vi "FPGA_R_ADC_W_DAC.vi"() -> ()   [LabVIEW 2019]
uses:
  <vilib>/rvi/Emulation/niFpgaGetClockAttributes.vi
  <vilib>/rvi/Emulation/niFpgaSctlEmulationGetInTimedLoop.vi
  <vilib>/rvi/Emulation/niFpgaEmulationReportErrorSimple.vi
  <vilib>/rvi/eio/common/nirviEmuTemplateMethod_errors.vi
  <vilib>/rvi/Emulation/niFpgaCriticalErrorInLSC.vi
  <vilib>/eio/EIONode/EIONode.xnode
panel:
  out "num refs":i16
  out "Tick Count(Ticks)":u32 caption="Encoder loop ticks"
  out "Encoder B Ref":bool
  out "Encoder A Ref":bool
  out "Encoder B":i32
  out "Encoder A":i32
  in  "stop 2":bool
  in  "Count(Ticks)":u32=800
  out "Data array":bool[](array[boolean])
  in  "stop":bool
  in  "DAC 3 write":bool[](array[boolean])=[FALSE, FALSE, FALSE, FALSE, FALSE, FALSE, FALSE, FALSE, FALSE, FALSE, FALSE, FALSE, FALSE, FALSE, FALSE, FALSE]
  in  "DAC 2 write":bool[](array[boolean])=[FALSE, FALSE, FALSE, FALSE, FALSE, FALSE, FALSE, FALSE, FALSE, FALSE, FALSE, FALSE, FALSE, FALSE, FALSE, FALSE]
  in  "DAC 1 write":bool[](array[boolean])=[FALSE, FALSE, FALSE, FALSE, FALSE, FALSE, FALSE, FALSE, FALSE, FALSE, FALSE, FALSE, FALSE, FALSE, FALSE, FALSE]
  out "ADC read":bool[](array[boolean])
  in  "ADC write":bool[](array[boolean])=[FALSE, FALSE, FALSE, FALSE, FALSE, TRUE, FALSE, FALSE, FALSE, FALSE, FALSE, FALSE, FALSE, FALSE, FALSE, FALSE]
  in  "Stop":bool
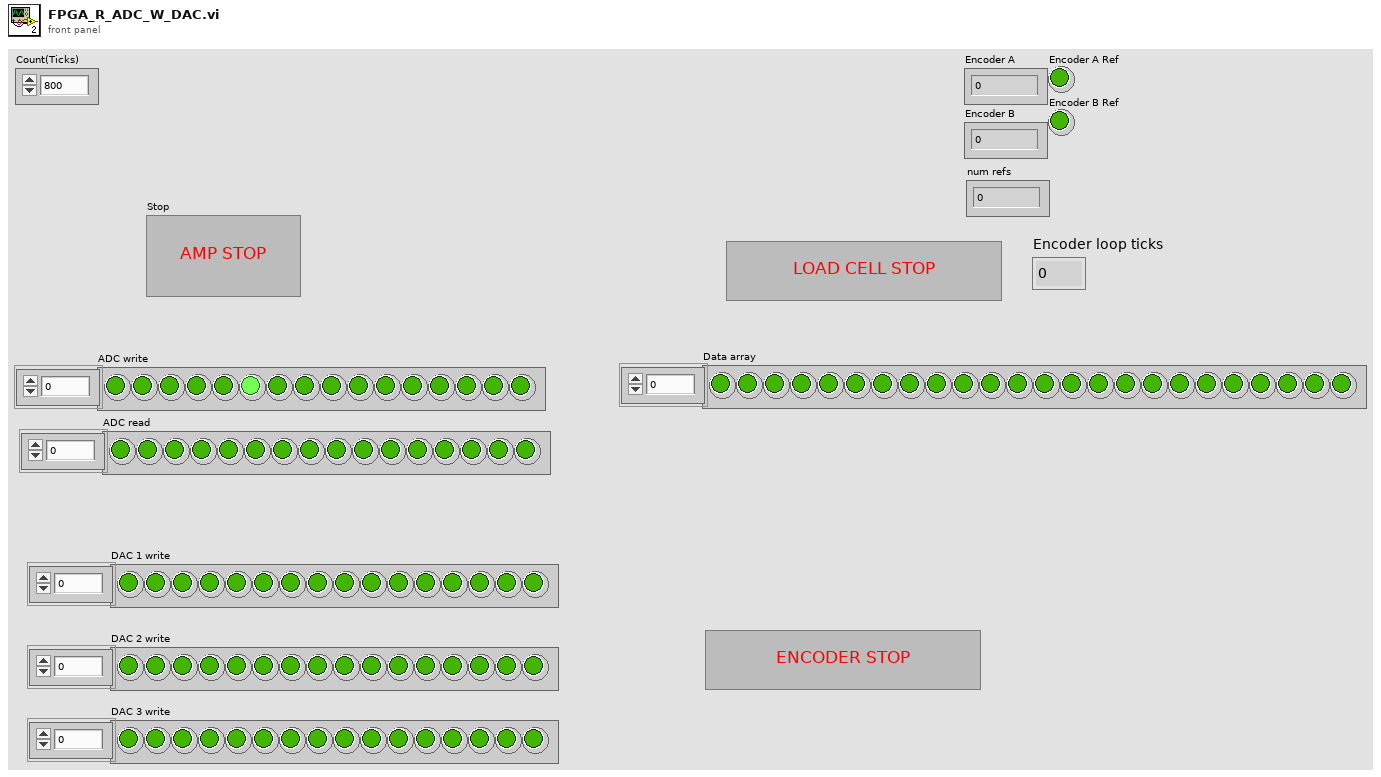
[diagram p1: front panel]
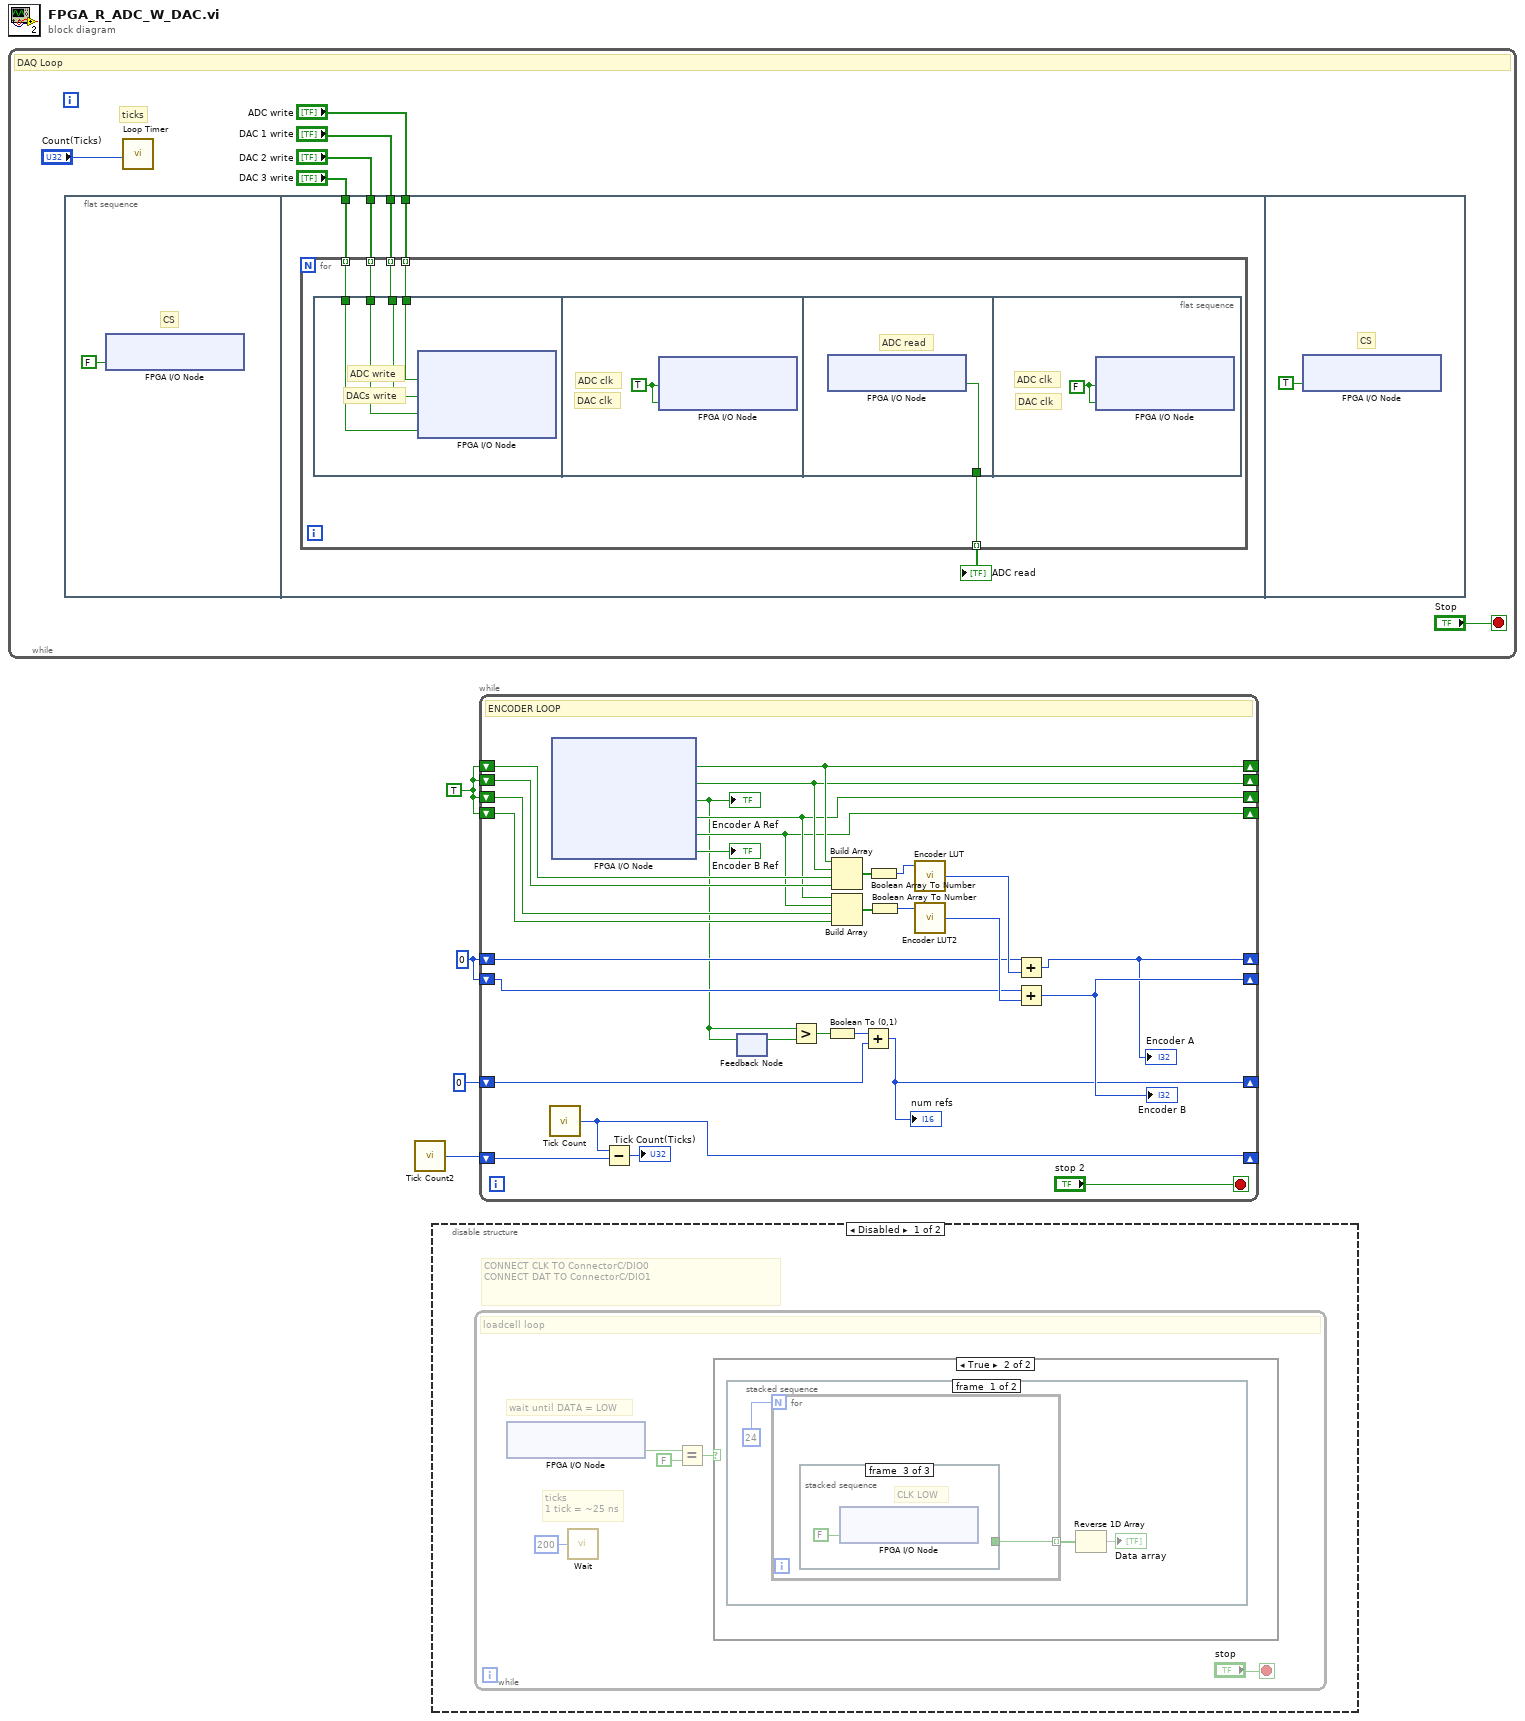
[diagram p0: block diagram]
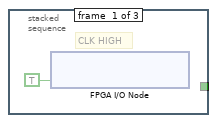
[diagram p3: hidden frame]
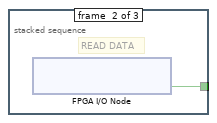
[diagram p4: hidden frame]
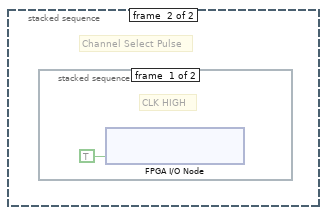
[diagram p5: hidden frame]
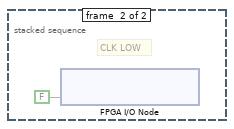
[diagram p6: hidden frame]
diagram:
  w3 = TRUE
  w4 = 0
  n1 = while {
    stop <- "Stop" stop-if-true
    # "ticks"
    # "DAQ Loop"
    n2 = flat-sequence {
      tunnel: "ADC write" -> [w16]
      tunnel: "DAC 1 write" -> [w14]
      tunnel: "DAC 2 write" -> [w13]
      tunnel: "DAC 3 write" -> [w12]
      frame #0 {
        # "CS"
        n3 = xnode "FPGA I/O Node"("ConnectorA/DIO4"=FALSE) -> ()  [unwired: 1 in, 1 out]
      }
      frame #1 {
        n4 = for {
          tunnel: w16 -> [w21] mode=indexing
          tunnel: [w20] -> w15 mode=indexing
          tunnel: w14 -> [w19] mode=indexing
          tunnel: w13 -> [w18] mode=indexing
          tunnel: w12 -> [w17] mode=indexing
          n5 = flat-sequence {
            tunnel: w21 -> [w25]
            tunnel: w19 -> [w24]
            tunnel: w18 -> [w23]
            tunnel: w17 -> [w22]
            tunnel: [w27] -> w20
            frame #0 {
              # "DACs write"
              # "ADC write"
              n6 = xnode "FPGA I/O Node"("ConnectorA/DIO2"=w25, "ConnectorA/DIO6"=w24, "ConnectorA/DIO7"=w23, "ConnectorA/DIO8"=w22) -> ()  [unwired: 4 in, 4 out]
            }
            frame #1 {
              w26 = TRUE ("ConnectorA/DIO3")
              # "DAC clk"
              # "ADC clk"
              n7 = xnode "FPGA I/O Node"("ConnectorA/DIO3"=w26, "ConnectorA/DIO5"=w26) -> ()  [unwired: 2 in, 2 out]
            }
            frame #2 {
              # "ADC read"
              n8 = xnode "FPGA I/O Node"() -> ("ConnectorA/DIO1"=w27:bool)  [unwired: 1 in, 1 out]
            }
            frame #3 {
              w28 = FALSE ("ConnectorA/DIO3")
              # "DAC clk"
              # "ADC clk"
              n9 = xnode "FPGA I/O Node"("ConnectorA/DIO3"=w28, "ConnectorA/DIO5"=w28) -> ()  [unwired: 2 in, 2 out]
            }
          }
        }
        "ADC read" <- w15
      }
      frame #2 {
        # "CS"
        n10 = xnode "FPGA I/O Node"("ConnectorA/DIO4"=TRUE) -> ()  [unwired: 1 in, 1 out]
      }
    }
    n11 = call "Loop Timer"("Count(Ticks)"="Count(Ticks)") -> ()  [unwired: 1 out]
  }
  n12 = call "Tick Count2"() -> ("Tick Count(Ticks)"=w2:u32)
  n13 = disable-structure shown="Disabled" {
    frame Disabled {
      # "CONNECT CLK TO ConnectorC/DIO0\nCONNECT DAT TO ConnectorC/DIO1"
      n14 = while {
        stop <- "stop" stop-if-true
        # "ticks\n1 tick = ~25 ns"
        # "wait until DATA = LOW"
        # "loadcell loop"
        n15 = xnode "FPGA I/O Node"() -> ("ConnectorC/DIO1"=w33:bool)  [unwired: 1 in, 1 out]
        n16 = call "Wait"("Count(Ticks)"=u32 200) -> ()  [unwired: 1 out]
        n17 = Equal?(x=w33, y=FALSE) -> (x = y?=w31:bool)
        n18 = case shown="True" w31 {
          frame False {
          }
          frame True {
            n19 = stacked-sequence {
              frame #0 {
                n20 = for {
                  N: 24 -> [_]
                  tunnel: [w38] -> w36 mode=indexing
                  n21 = stacked-sequence {
                    tunnel: [_ w40 _] -> w38
                    frame #0 {
                      # "CLK HIGH"
                      n22 = xnode "FPGA I/O Node"("ConnectorC/DIO0"=TRUE ("ConnectorB/DIO0")) -> ()  [unwired: 1 in, 1 out]
                    }
                    frame #1 {
                      # "READ DATA"
                      n23 = xnode "FPGA I/O Node"() -> ("ConnectorC/DIO1"=w40:bool)  [unwired: 1 in, 1 out]
                    }
                    frame #2 {
                      # "CLK LOW"
                      n24 = xnode "FPGA I/O Node"("ConnectorC/DIO0"=FALSE ("ConnectorB/DIO0")) -> ()  [unwired: 1 in, 1 out]
                    }
                  }
                }
                n25 = Reverse 1D Array(array=w36) -> (reversed array=→"Data array":bool[])
              }
              frame #1 {
                # "Channel Select Pulse"
                n26 = stacked-sequence {
                  frame #0 {
                    # "CLK HIGH"
                    n27 = xnode "FPGA I/O Node"("ConnectorC/DIO0"=TRUE ("ConnectorB/DIO0")) -> ()  [unwired: 1 in, 1 out]
                  }
                  frame #1 {
                    # "CLK LOW"
                    n28 = xnode "FPGA I/O Node"("ConnectorC/DIO0"=FALSE ("ConnectorB/DIO0")) -> ()  [unwired: 1 in, 1 out]
                  }
                }
              }
            }
          }
        }
      }
    }
    frame Enabled {
    }
  }
  n29 = while {
    shift-right: [w53] -> _
    shift-left: w4 -> [w56]
    shift-right: [w61] -> _
    shift-left: w3 -> [w71]
    shift-right: [w60] -> _
    shift-left: w3 -> [w66]
    shift-right: [w59] -> _
    shift-left: w3 -> [w65]
    shift-right: [w58] -> _
    shift-left: w3 -> [w64]
    shift-right: [w54] -> _
    shift-left: w4 -> [w55]
    shift-right: [w51] -> _
    shift-left: w2 -> [w52]
    shift-right: [w44] -> _
    shift-left: i16 0 -> [w45]
    stop <- "stop 2" stop-if-true
    # "ENCODER LOOP"
    n30 = call "Tick Count"() -> ("Tick Count(Ticks)"=w51:u32)
    n31 = xnode "FPGA I/O Node"() -> ("ConnectorA/DIO9"=w61:bool, "ConnectorA/DIO10"=w60:bool, "ConnectorA/DIO11"=w49:bool, "ConnectorA/DIO13"=w59:bool, "ConnectorA/DIO14"=w58:bool, "ConnectorA/DIO12"=→"Encoder B Ref":bool)  [unwired: 6 in, 6 out]
    "Encoder A Ref" <- w49
    n32 = Subtract(x=w51, y=w52) -> (x-y=→"Tick Count(Ticks)":u32)
    n33 = feedback-in #1(w49) -> ()
    n34 = feedback #1() -> (w48:bool)  [unwired: 1 in]
    n35 = Greater?(x=w49, y=w48) -> (0:w47:bool)
    n36 = Boolean To (0,1)(Boolean=w47) -> (0, 1=w46:i16)
    n37 = Build Array(w61, w60, w71, w66) -> (w69:bool[])
    n38 = Build Array(w59, w58, w65, w64) -> (w70:bool[])
    n39 = Add(x=w46, y=w45) -> (x+y=w44:i16)
    "num refs" <- w44
    n40 = Boolean Array To Number(Boolean array=w69) -> (number=w68:u8)
    n41 = Boolean Array To Number(Boolean array=w70) -> (number=w67:u8)
    n42 = call "Encoder LUT"("address"=w68) -> ("data out"=w63:i32)  [unwired: 8 in]
    n43 = call "Encoder LUT2"("address"=w67) -> ("data out"=w62:i32)  [unwired: 8 in]
    n44 = Add(x=w56, y=w63) -> (x+y=w53:i32)
    "Encoder A" <- w53
    n45 = Add(x=w55, y=w62) -> (x+y=w54:i32)
    "Encoder B" <- w54
  }
